vi "Inovance_Get_Frame_SubVI.vi"(8 "error in (no error)":errorcluster, 9 "Session Out in":T1, 10 "BCG Values":T3, 11 "Refnum in":T2) -> (0 "error out":errorcluster, 3 "Refnum out":T1)   [LabVIEW 2023, in "Inovance_Camera.lvlib"]
uses:
  <vilib>/vision/Image Controls.llb/IMAQ Image.ctl
  <vilib>/userDefined/High Color/IMAQdx.ctl
  Inovance_Camera.lvlib
  <vilib>/vision/driver/NI_Vision_Acquisition_Software.lvlib
  <vilib>/vision/NI_Vision_Development_Module.lvlib
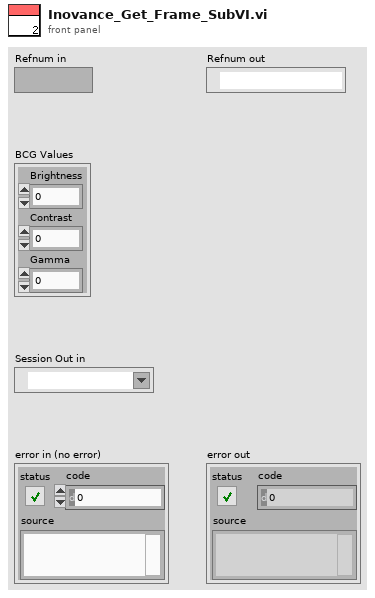
[diagram p1: front panel]
types:
  T1 = typedef "IMAQdx.ctl" = refnum<k21>
  T2 = typedef "IMAQ Image.ctl" = refnum<image>
  T3 = cluster{"Brightness":sgl, "Contrast":sgl, "Gamma":sgl}
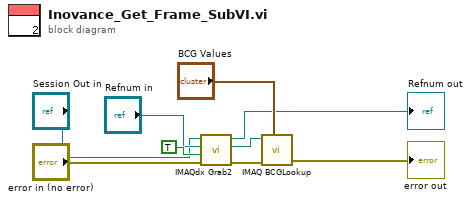
[diagram p0: block diagram]
diagram:
  n1 = call <vilib>:"IMAQdx Grab2.vi"("error in"="error in (no error)", "Wait for Next Buffer? (Yes)"=TRUE, "Image In"="Refnum in", "Session In"="Session Out in") -> ("error out"=w8:errorcluster, "Image Out"=w7:T2, "Session Out"=→"Refnum out":T1)  [unwired: 4 in, 1 out]
  n2 = call "IMAQ BCGLookup"("Image Src"=w7, "BCG Values"="BCG Values", "error in (no error)"=w8) -> ("error out"=→"error out":errorcluster)  [unwired: 4 in, 1 out]
